vi "例程19-写入文本文件.vi"() -> ()   [LabVIEW 2016]
panel:
  out "数组":string[](array[string])
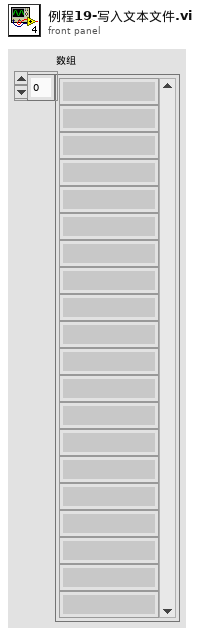
[diagram p1: front panel]
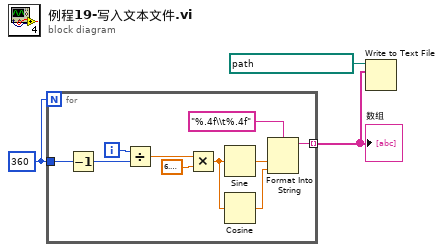
[diagram p0: block diagram]
diagram:
  w2 = 360
  n1 = for {
    N: w2 -> [_]
    tunnel: [w11] -> w1 mode=indexing
    tunnel: w2 -> [w9]
    i -> [w13]
    n2 = Decrement(x=w9) -> (x-1=w10:i32)
    n3 = Divide(x=w13, y=w10) -> (x/y=w8:dbl)
    n4 = Multiply(x=w8, y=6.283185307179586) -> (x*y=w4:dbl)
    n5 = Sine(x=w4) -> (sin(x)=w5:dbl)
    n6 = Cosine(x=w4) -> (cos(x)=w6:dbl)
    n7 = Format Into String(format string="%.4f\\t%.4f" ("格式字符串"), w5, w6) -> (resulting string=w11:string)  [unwired: 2 in, 1 out]
  }
  "数组" <- w1
  n8 = Write to Text File(file (use dialog)=path "D:/文本文件写入.csv" ("文件（使用对话框）"), text=w1) -> ()  [unwired: 2 in, 3 out]
